vi "go to desired page.vi"(0 "VISA in":refnum<visa-resource-name>, 7 "Set Cluster":T1={"set index"=0, "set Screen"="Main Menu", "set subpage"=0, "set column"=0, "Group"="", "Crate"=0}, 11 "error in":errorcluster) -> (4 "VISA out":refnum<visa-resource-name>, 6 "Location Cluster out":T2, 8 "Display array":string[][](array[string]), 15 "error out":errorcluster)   [LabVIEW 2018]
uses:
  location cluster.ctl
  set location.ctl
  CAEN globals.vi
panel:
  out "num pages":i32
  # "crate channel screen subpage column"
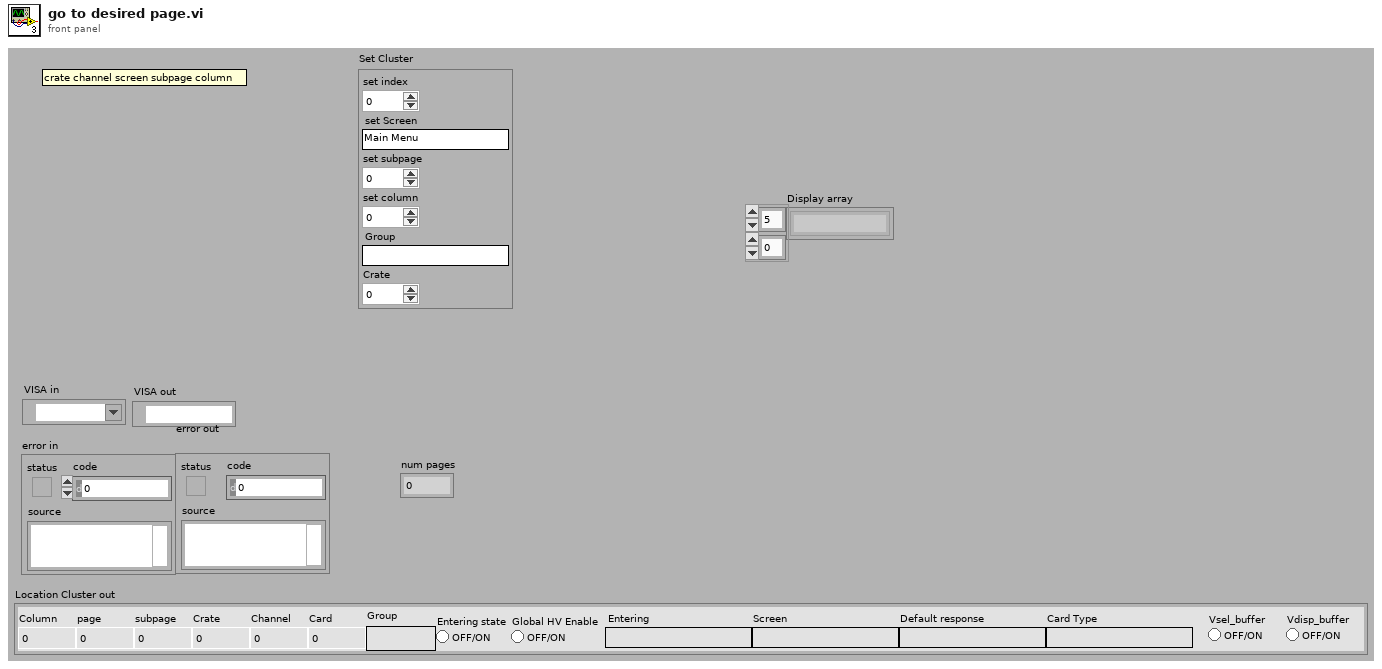
[diagram p1: front panel]
types:
  T1 = typedef "set location.ctl" = cluster{"set index":i32, "set Screen":string, "set subpage":i32, "set column":i32, "Group":string, "Crate":i32}
  T2 = typedef "location cluster.ctl" = cluster{"Column":i32, "Card Type":string, "Channel":i32, "Card":i32, "Default response":string, "Entering":string, "Entering state":bool, "subpage":i32, "page":i32, "Crate":i32, "Screen":string, "Group":string, "Global HV Enable":bool, "Vsel_buffer":bool, "Vdisp_buffer":bool}
  T3 = cluster{"set crate":i32, "set channel":i32, "Property":string}
  T4 = cluster{"set Screen":string, "set subpage":i32, "set column":i32}
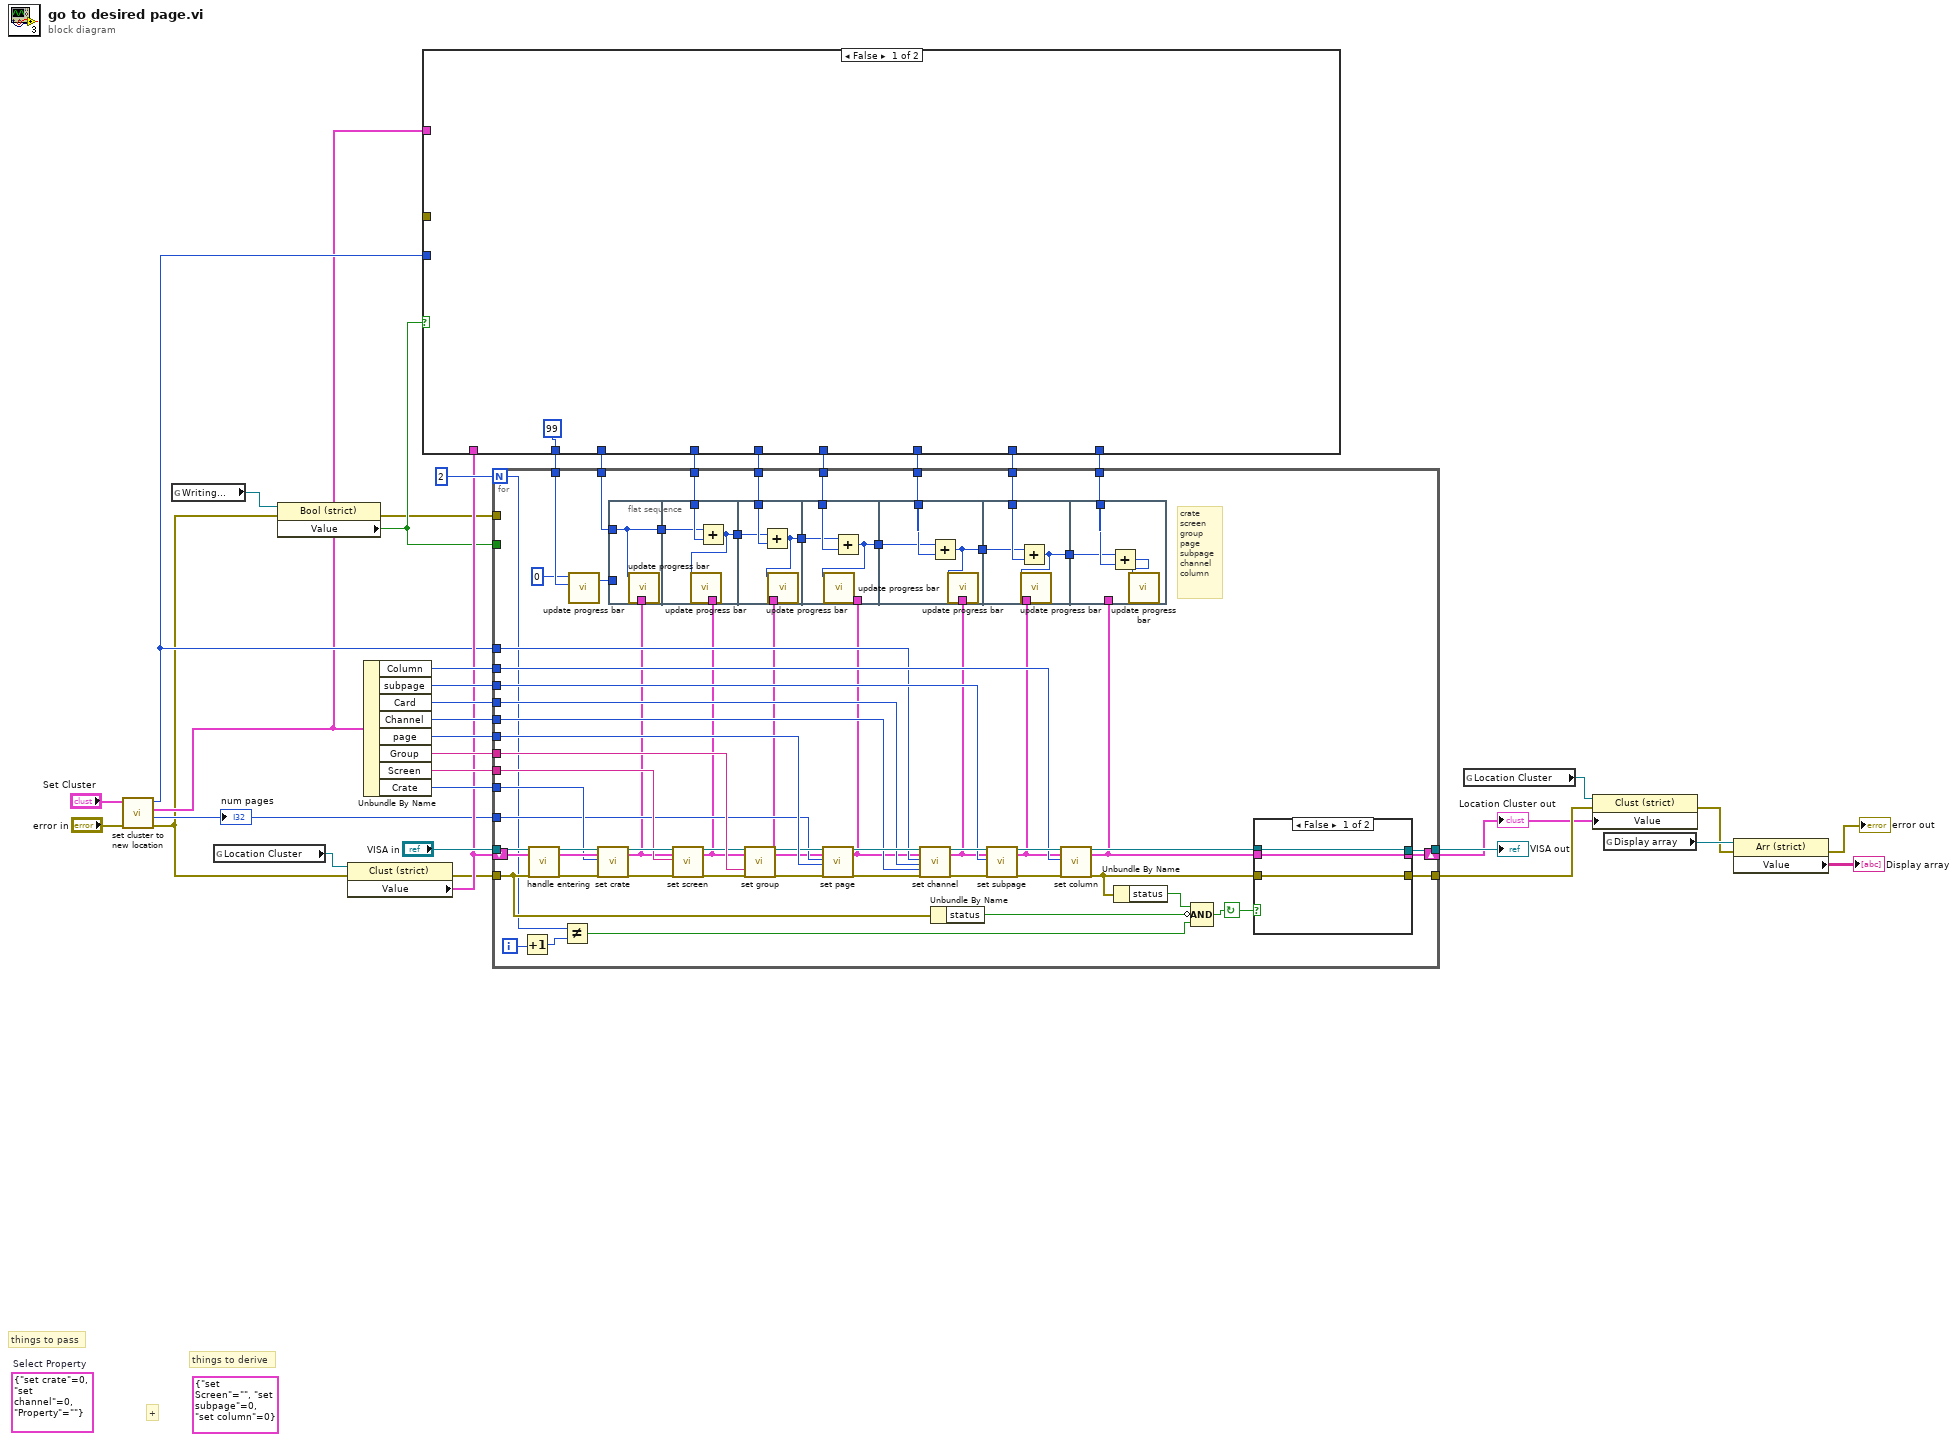
[diagram p0: block diagram]
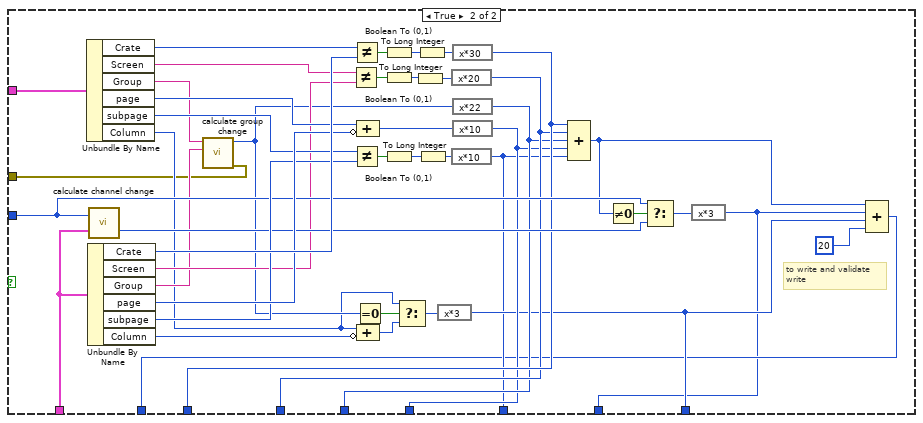
[diagram p2: hidden frame]
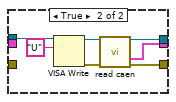
[diagram p3: hidden frame]
diagram:
  (unwired) T3 {"set crate"=0, "set channel"=0, "Property"=""}  # Select Property
  (unwired) T4 {"set Screen"="", "set subpage"=0, "set column"=0} ("Set Cluster 2")
  # "+"
  # "things to pass"
  # "things to derive"
  n1 = call "set cluster to new location.vi"("error in"="error in", "Set Cluster"="Set Cluster") -> ("error out"=w4:errorcluster, "num pages"=w5:i32, "Location Cluster out"=w7:T2, "set index"=w17:i32)  [unwired: 6 in]
  "num pages" <- w5
  n2 = global read "CAEN globals.vi" "Writing..."() -> (w6:refnum<vi>)
  n3 = global read "CAEN globals.vi" "Location Cluster"() -> (w31:refnum<vi>)
  n4 = property class="Bool (strict)"(reference=w6, error in=w4) -> (error out=w2:errorcluster, "Value"=w3:bool)  [unwired: 1 out]
  n5 = property class="Clust (strict)"(reference=w31, error in=w4) -> (error out=w12:errorcluster, "Value"=w18:T2)  [unwired: 1 out]
  n6 = Unbundle By Name(w7) -> ("Column"=w30:i32, "subpage"=w29:i32, "Card"=w20:i32, "Channel"=w21:i32, "page"=w28:i32, "Group"=w24:string, "Screen"=w27:string, "Crate"=w26:i32)
  n7 = case shown="False" w3 {
    tunnel: w7 -> [_ w82]
    tunnel: w18 -> [_ w74]
    tunnel: w17 -> [_ w67]
    tunnel: [_ w56] -> w16
    tunnel: [_ w55] -> w15
    tunnel: [_ w54] -> w14
    tunnel: [_ w53] -> w13
    tunnel: [_ w52] -> w11
    tunnel: [_ w51] -> w10
    tunnel: [99 w50] -> w9
    tunnel: [_ w47] -> w8
    tunnel: [_ w46] -> _
    frame False {
    }
    frame True {
      # "to write and validate\nwrite"
      n8 = Unbundle By Name(w82) -> ("Crate"=w81:i32, "Screen"=w79:string, "Group"=w66:string, "page"=w78:i32, "subpage"=w76:i32, "Column"=w59:i32)
      n9 = Unbundle By Name(w74) -> ("Crate"=w80:i32, "Screen"=w65:string, "Group"=w64:string, "page"=w77:i32, "subpage"=w75:i32, "Column"=w63:i32)
      n10 = call "calculate channel change.vi"("set index"=w67, "Location Cluster in"=w74) -> ("rows difference"=w68:i32)  [unwired: 15 in, 2 out]
      n11 = call "calculate group change.vi"("Current group"=w64, "Set group"=w66) -> ("error out"=w46:errorcluster, "num changes"=w61:i32)  [unwired: 6 in, 2 out]
      n12 = Not Equal?(x=w79, y=w65) -> (x != y?=w71:bool)
      n13 = Not Equal?(x=w81, y=w80) -> (x != y?=w73:bool)
      n14 = Not Equal?(x=w76, y=w75) -> (x != y?=w72:bool)
      n15 = Equal To 0?(x=w61) -> (x = 0?=w62:bool)
      n16 = Compound Arithmetic op=ADD(w78, invert w77) -> (w70:i32)
      n17 = Compound Arithmetic op=ADD(w59, invert w63) -> (w60:i32)
      n18 = Boolean To (0,1)(Boolean=w73) -> (0, 1=w40:i16)
      n19 = Boolean To (0,1)(Boolean=w71) -> (0, 1=w43:i16)
      n20 = Boolean To (0,1)(Boolean=w72) -> (0, 1=w44:i16)
      n21 = Select(t=w59, s=w62, f=w60) -> (s? t:f=w58:i32)
      n22 = To Long Integer(number=w43) -> (32bit integer=w42:i32)
      n23 = To Long Integer(number=w40) -> (32bit integer=w41:i32)
      n24 = To Long Integer(number=w44) -> (32bit integer=w45:i32)
      n25 = expression code="x*3"(w58) -> (w52:i32)
      n26 = expression code="x*20"(w42) -> (w55:i32)
      n27 = expression code="x*10"(w45) -> (w51:i32)
      n28 = expression code="x*30"(w41) -> (w56:i32)
      n29 = expression code="x*22"(w61) -> (w54:i32)
      n30 = expression code="x*10"(w70) -> (w53:i32)
      n31 = Compound Arithmetic op=ADD(w56, w55, w54, w53, w51) -> (w57:i32)
      n32 = Not Equal To 0?(x=w57) -> (x != 0?=w69:bool)
      n33 = Select(t=w67, s=w69, f=w68) -> (s? t:f=w48:i32)
      n34 = expression code="x*3"(w48) -> (w47:i32)
      n35 = Compound Arithmetic op=ADD(w57, w47, w52, 20 ("value")) -> (w50:i32)
    }
  }
  n36 = for {
    N: 2 -> [w86]
    tunnel: w30 -> [w133]
    tunnel: w29 -> [w132]
    tunnel: w28 -> [w131]
    tunnel: w27 -> [w130]
    tunnel: w26 -> [w129]
    tunnel: w24 -> [w128]
    tunnel: w21 -> [w123]
    tunnel: w20 -> [w122]
    tunnel: w5 -> [w121]
    tunnel: w17 -> [w120]
    shift-right: [w87] -> w1
    shift-left: w18 -> [w134]
    tunnel: "VISA in" -> [w140]
    tunnel: [w114] -> w38
    tunnel: w12 -> [w99]
    tunnel: [w115] -> w23
    tunnel: w9 -> [w97]
    tunnel: w16 -> [w112]
    tunnel: w15 -> [w111]
    tunnel: w14 -> [w110]
    tunnel: w13 -> [w109]
    tunnel: w10 -> [w108]
    tunnel: w8 -> [w107]
    tunnel: w11 -> [w98]
    tunnel: w3 -> [_]
    tunnel: w2 -> [_]
    i -> [w84]
    stop <- w113 continue-if-true
    # "crate\nscreen\ngroup\npage\nsubpage\nchannel\ncolumn"
    n37 = Increment(x=w84) -> (x+1=w83:i32)
    n38 = call "handle entering.vi"("VISA in"=w140, "Current location"=w134, "error in"=w99) -> ("VISA out"=w139:refnum<visa-resource-name>, "Location Cluster"=w138:T2, "error out"=w137:errorcluster)  [unwired: 14 in]
    n39 = Not Equal?(x=w86, y=w83) -> (x != y?=w85:bool)
    n40 = call "update progress bar.vi"("Max"=w97, "Progress"=0) -> ("Write progress"=w89:u8)  [unwired: 5 in]
    n41 = call "set crate.vi"("VISA in"=w139, "Location Cluster in"=w138, "set crate"=w129, "error in"=w137) -> ("VISA out"=w136:refnum<visa-resource-name>, "Location Cluster out"=w106:T2, "error out"=w135:errorcluster)  [unwired: 13 in]
    n42 = flat-sequence {
      tunnel: w112 -> [w146]
      tunnel: [w146] -> w96
      tunnel: w106 -> [_]
      tunnel: w89 -> [_]
      tunnel: w96 -> [w148]
      tunnel: w111 -> [w149]
      tunnel: [w147] -> w95
      tunnel: w105 -> [_]
      tunnel: w95 -> [w151]
      tunnel: w110 -> [w152]
      tunnel: [w150] -> w94
      tunnel: w104 -> [_]
      tunnel: w94 -> [w154]
      tunnel: w109 -> [w155]
      tunnel: [w153] -> w93
      tunnel: w103 -> [_]
      tunnel: w93 -> [w157]
      tunnel: w108 -> [w158]
      tunnel: [w156] -> w92
      tunnel: w102 -> [_]
      tunnel: w92 -> [w160]
      tunnel: w107 -> [w161]
      tunnel: w101 -> [_]
      tunnel: [w159] -> w91
      tunnel: w100 -> [_]
      tunnel: w91 -> [w163]
      tunnel: w98 -> [w164]
      frame #0 {
        n43 = call "update progress bar.vi"("Progress"=w146) -> ()  [unwired: 6 in, 1 out]
      }
      frame #1 {
        n44 = Add(x=w148, y=w149) -> (x+y=w147:i32)
        n45 = call "update progress bar.vi"("Progress"=w147) -> ()  [unwired: 6 in, 1 out]
      }
      frame #2 {
        n46 = Add(x=w151, y=w152) -> (x+y=w150:i32)
        n47 = call "update progress bar.vi"("Progress"=w150) -> ()  [unwired: 6 in, 1 out]
      }
      frame #3 {
        n48 = Add(x=w154, y=w155) -> (x+y=w153:i32)
        n49 = call "update progress bar.vi"("Progress"=w153) -> ()  [unwired: 6 in, 1 out]
      }
      frame #4 {
        n50 = Add(x=w157, y=w158) -> (x+y=w156:i32)
        n51 = call "update progress bar.vi"("Progress"=w156) -> ()  [unwired: 6 in, 1 out]
      }
      frame #5 {
        n52 = Add(x=w160, y=w161) -> (x+y=w159:i32)
        n53 = call "update progress bar.vi"("Progress"=w159) -> ()  [unwired: 6 in, 1 out]
      }
      frame #6 {
        n54 = Add(x=w163, y=w164) -> (x+y=w162:i32)
        n55 = call "update progress bar.vi"("Progress"=w162) -> ()  [unwired: 6 in, 1 out]
      }
    }
    n56 = call "set screen.vi"("VISA in"=w136, "Location Cluster in"=w106, "set Screen"=w130, "error in"=w135) -> ("VISA out"=w127:refnum<visa-resource-name>, "Location Cluster out"=w105:T2, "error out"=w125:errorcluster)  [unwired: 13 in]
    n57 = call "set group.vi"("VISA in"=w127, "Location Cluster in"=w105, "Group"=w128, "error in (no error)"=w125) -> ("VISA out"=w126:refnum<visa-resource-name>, "Location Cluster out"=w104:T2, "error out"=w124:errorcluster)  [unwired: 13 in]
    n58 = call "set page.vi"("VISA in"=w126, "Location Cluster in"=w104, "num pages"=w121, "set page"=w131, "error in"=w124) -> ("VISA out"=w141:refnum<visa-resource-name>, "Location Cluster out"=w103:T2, "error out"=w119:errorcluster)  [unwired: 12 in]
    n59 = call "set channel.vi"("VISA in"=w141, "Location Cluster in"=w103, "set row"=w120, "set card"=w122, "set channel"=w123, "error in"=w119) -> ("VISA out"=w145:refnum<visa-resource-name>, "Location Cluster out"=w102:T2, "error out"=w144:errorcluster)  [unwired: 11 in]
    n60 = Unbundle By Name(w99) -> ("status"=w117:bool)
    n61 = call "set subpage.vi"("VISA in"=w145, "Location Cluster in"=w102, "set subpage"=w132, "error in"=w144) -> ("VISA out"=w143:refnum<visa-resource-name>, "Location Cluster out"=w101:T2, "error out"=w142:errorcluster)  [unwired: 13 in]
    n62 = call "set column.vi"("VISA in"=w143, "Location Cluster in"=w101, "set column"=w133, "error in"=w142) -> ("VISA out"=w116:refnum<visa-resource-name>, "Location Cluster out"=w100:T2, "error out"=w88:errorcluster)  [unwired: 13 in]
    n63 = Unbundle By Name(w88) -> ("status"=w118:bool)
    n64 = Compound Arithmetic op=AND(w118, invert w117, w85) -> (w113:bool)
    n65 = case shown="False" w113 {
      tunnel: w116 -> [w165 w174]
      tunnel: w88 -> [w166 _]
      tunnel: [w166 w170] -> w115
      tunnel: [w167 w169] -> w87
      tunnel: w100 -> [w167 _]
      tunnel: [w165 w168] -> w114
      frame False {
      }
      frame True {
        n66 = VISA Write(VISA resource name=w174, write buffer="U") -> (VISA resource name out=w172:refnum<visa-resource-name>, error out=w171:errorcluster)  [unwired: 1 in, 1 out]
        n67 = call "read caen.vi"("VISA in"=w172, "error in"=w171) -> ("VISA out"=w168:refnum<visa-resource-name>, "Location Cluster"=w169:T2, "error out"=w170:errorcluster)  [unwired: 8 in, 3 out]
      }
    }
  }
  "Location Cluster out" <- w1
  "VISA out" <- w38
  n68 = global read "CAEN globals.vi" "Location Cluster"() -> (w33:refnum<vi>)
  n69 = property class="Clust (strict)"(reference=w33, error in=w23, "Value"=w1) -> (error out=w32:errorcluster)  [unwired: 1 out]
  n70 = global read "CAEN globals.vi" "Display array"() -> (w36:refnum<vi>)
  n71 = property class="Arr (strict)"(reference=w36, error in=w32) -> (error out=→"error out":errorcluster, "Value"=→"Display array":string[][])  [unwired: 1 out]
